vi "Receive Messages.vi"(8 "error in":errorcluster, 10 "Sender ID":string, 11 "PCAN in":refnum<class "PCAN.lvclass">) -> (0 "error out":errorcluster, 2 "Messages":refnum<class "IMessage.lvclass">[](array[class]), 3 "PCAN out":refnum<class "PCAN.lvclass">)   [LabVIEW 2024, in "PCAN.lvlib" / "PCAN.lvclass"]
uses:
  PCAN.lvclass
  PCAN.lvclass/PCAN.ctl
  CAN Message/CAN Message.lvclass
  Source/Interfaces/IMessage/IMessage.lvclass
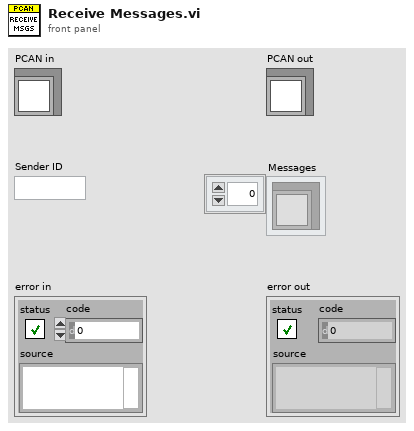
[diagram p1: front panel]
types:
  T1 = typedef "TPCANHandle.ctl" = enum16{"PCAN_NONEBUS  0x000", "PCAN_ISABUS1  0x21", "PCAN_ISABUS2  0x22", "PCAN_ISABUS3  0x23", "PCAN_ISABUS4  0x24", "PCAN_ISABUS5  0x25", "PCAN_ISABUS6  0x26", "PCAN_ISABUS7  0x27", "PCAN_ISABUS8  0x28", "PCAN_DNGBUS1  0x31", "PCAN_PCIBUS1  0x41", "PCAN_PCIBUS1  0x42", "PCAN_PCIBUS1  0x43", "PCAN_PCIBUS1  0x44", "PCAN_PCIBUS1  0x45", "PCAN_PCIBUS1  0x46", "PCAN_PCIBUS1  0x47", "PCAN_PCIBUS1  0x48", "PCAN_PCIBUS1  0x409", "PCAN_PCIBUS1  0x40A", "PCAN_PCIBUS1  0x40B", "PCAN_PCIBUS1  0x40C", "PCAN_PCIBUS1  0x40D", "PCAN_PCIBUS1  0x40E", "PCAN_PCIBUS1  0x40F", "PCAN_PCIBUS1  0x410", "PCAN_USBBUS1  0x51", "PCAN_USBBUS2  0x52", "PCAN_USBBUS3  0x53", "PCAN_USBBUS4  0x54", "PCAN_USBBUS5  0x55", "PCAN_USBBUS6  0x56", "PCAN_USBBUS7  0x57", "PCAN_USBBUS8  0x58", "PCAN_USBBUS9  0x509", "PCAN_USBBUS10  0x50A", "PCAN_USBBUS11  0x50B", "PCAN_USBBUS12  0x50C", "PCAN_USBBUS13  0x50D", "PCAN_USBBUS14  0x50E", "PCAN_USBBUS15  0x50F", "PCAN_USBBUS16  0x510", "PCAN_PCCBUS1  0x61", "PCAN_PCCBUS2  0x62", "PCAN_LANBUS1  0x801", "PCAN_LANBUS2  0x802", "PCAN_LANBUS3  0x803", "PCAN_LANBUS4  0x804", "PCAN_LANBUS5  0x805", "PCAN_LANBUS6  0x806", "PCAN_LANBUS7  0x807", "PCAN_LANBUS8  0x808", "PCAN_LANBUS9  0x809", "PCAN_LANBUS10  0x80A", "PCAN_LANBUS11  0x80B", "PCAN_LANBUS12  0x80C", "PCAN_LANBUS13  0x80D", "PCAN_LANBUS14  0x80E", "PCAN_LANBUS15  0x80F", "PCAN_LANBUS16  0x810"}
  T2 = typedef "TPCANTimestamp.ctl" = cluster{"millis overflow":u16, "millis ":u32, "micros":u16}
  T3 = typedef "CAN MSG Cluster.ctl" = cluster{"ID":u32, "MSG type":u8, "DLC":u8, "DATA":u8[]}
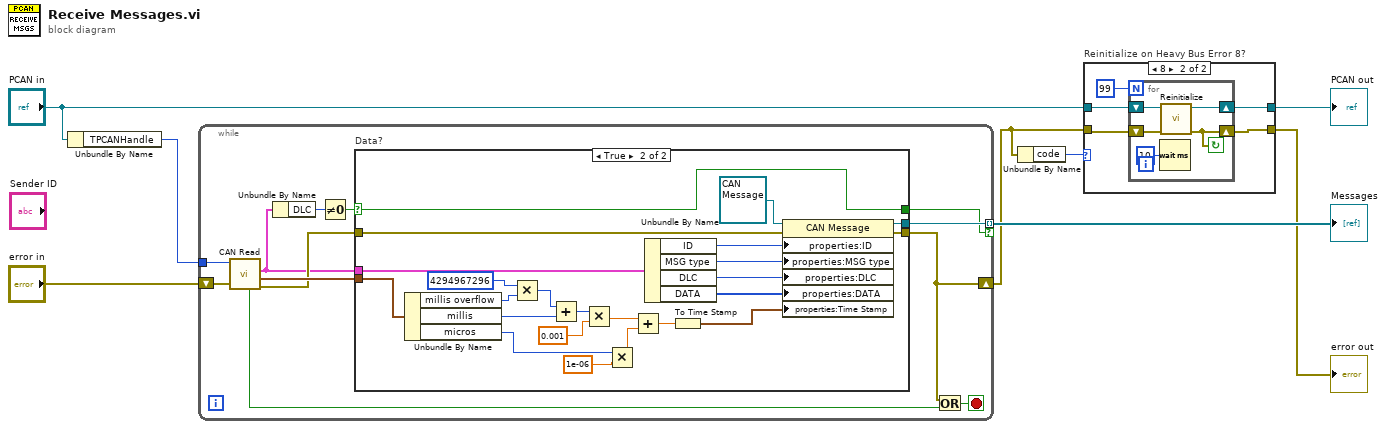
[diagram p0: block diagram]
diagram:
  n1 = Unbundle By Name("PCAN in") -> ("TPCANHandle"=w8:T1)
  n2 = while {
    tunnel: w8 -> [w20]
    tunnel: [w17] -> w6 mode=indexing if=w9
    shift-right: [w14] -> w4
    shift-left: "error in" -> [w19]
    stop <- w15 stop-if-true
    n3 = call <instrlib>:"CAN Read.vi"("error in (no error)"=w19, "TPCANHandle"=w20) -> ("error out"=w16:errorcluster, "TPCANTimestamp out"=w18:T2, "CAN_Message out"=w12:T3, "rcv queue empty"=w13:bool)  [unwired: 5 in, 1 out]
    n4 = Unbundle By Name(w12) -> ("DLC"=w10:u8)
    n5 = Not Equal To 0?(x=w10) -> (x != 0?=w11:bool)
    n6 = case "Data?" shown="True" w11 {
      selector: w11 -> [w21 w23]
      tunnel: w18 -> [_ w45]
      tunnel: w12 -> [_ w44]
      tunnel: [_ w31] -> w17
      tunnel: w16 -> [w22 w25]
      tunnel: [w22 w24] -> w14
      tunnel: [w21 w23] -> w9
      frame False {
      }
      frame True {
        n7 = Unbundle By Name(w45) -> ("millis overflow"=w35:u16, "millis"=w38:u32, "micros"=w37:u16)
        n8 = Multiply(x=u64 4294967296, y=w35) -> (x*y=w33:u64)
        n9 = Add(x=w33, y=w38) -> (x+y=w34:u64)
        n10 = Multiply(x=w34, y=0.001) -> (x*y=w40:dbl)
        n11 = Multiply(x=w37, y=1e-06) -> (x*y=w41:dbl)
        n12 = Add(x=w40, y=w41) -> (x+y=w39:dbl)
        n13 = Unbundle By Name(w44) -> ("ID"=w30:u32, "MSG type"=w29:u8, "DLC"=w28:u8, "DATA"=w27:u8[])
        n14 = To Time Stamp(1:w39) -> (0:w26:timestamp)
        n15 = property class="CAN Message"(reference=refnum<class "CAN Message.lvclass"> refnum ("PCAN.lvlib:CAN Message"), error in=w25, "properties:ID"=w30, "properties:MSG type"=w29, "properties:DLC"=w28, "properties:DATA"=w27, "properties:Time Stamp"=w26) -> (reference out=w31:refnum<class "CAN Message.lvclass">, error out=w24:errorcluster)
      }
    }
    n16 = Or(x=w14, y=w13) -> (x .or. y?=w15:bool)
  }
  "Messages" <- w6
  n17 = Unbundle By Name(w4) -> ("code"=w3:i32)
  n18 = case "Reinitialize on Heavy Bus Error 8?" shown="8" w3 {
    tunnel: [w47 w52] -> w1
    tunnel: w4 -> [w47 w48]
    tunnel: "PCAN in" -> [w46 w51]
    tunnel: [w46 w50] -> w2
    frame Default {
    }
    frame 8 {
      n19 = for {
        N: 99 -> [_]
        shift-right: [w56] -> w50
        shift-left: w51 -> [w57]
        shift-right: [w55] -> w52
        shift-left: w48 -> [w53]
        stop <- w55 continue-if-true
        n20 = Wait (ms)(milliseconds to wait=u32 10) -> ()  [unwired: 1 out]
        n21 = call "Reinitialize.vi"("error in"=w53, "PCAN in"=w57) -> ("error out"=w55:errorcluster, "PCAN out"=w56:refnum<class "PCAN.lvclass">)  [unwired: 8 in]
      }
    }
  }
  "error out" <- w1
  "PCAN out" <- w2
